vi "Read Params from INI Section.vi"(8 "error in (no error)":errorcluster, 9 "Parameters In":variant, 10 "Refnum in":T1, 11 "Analyze Fluence in":refnum<class "Analyze Fluence.lvclass">) -> (0 "error out":errorcluster, 1 "Parameters Out":variant, 2 "Refnum out":T1, 3 "Analyze Fluence out":refnum<class "Analyze Fluence.lvclass">)   [LabVIEW 2020, in "Analyze.lvlib" / "Analyze Fluence.lvclass"]
uses:
  Analyze Fluence.lvclass
  <vilib>/Utility/config.llb/Config Data RefNum.ctl
  <vilib>/Utility/config.llb/Read Key (Double).vi
  <vilib>/Utility/config.llb/Read Key (I32).vi
  <vilib>/Utility/config.llb/NI_LVConfig.lvlib
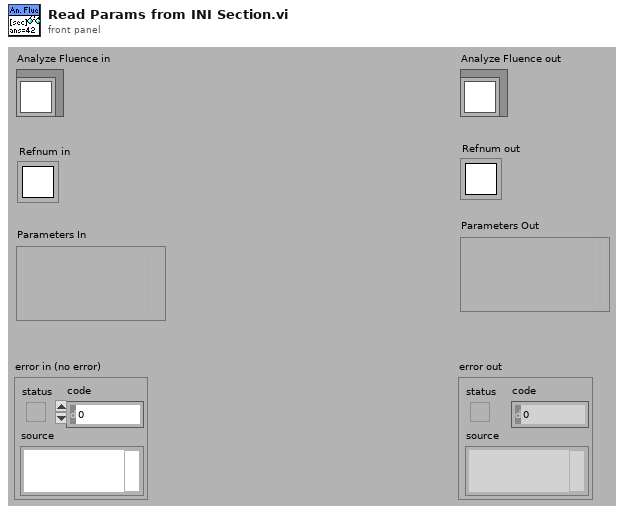
[diagram p1: front panel]
types:
  T1 = typedef "NI_LVConfig.lvlib/Config Data RefNum.ctl" = refnum<k1>
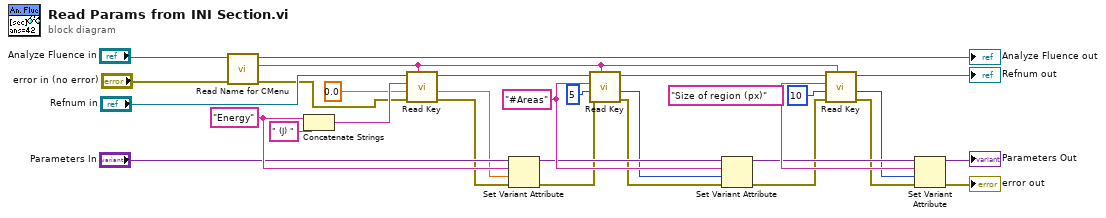
[diagram p0: block diagram]
diagram:
  w30 = "Size of region (px)" ("name")
  w27 = "#Areas" ("name")
  w23 = "Energy" ("name")
  n1 = call-dynamic "Read Name for CMenu.vi"("error in (no error)"="error in (no error)", "Analyze BaseClass in"="Analyze Fluence in") -> ("error out"=w18:errorcluster, "Name for Context menu"=w1:string, "Analyze BaseClass out"=→"Analyze Fluence out":refnum<class "Analyze Fluence.lvclass">)  [unwired: 7 in]
  n2 = Concatenate Strings(w23, " (J) " ("string")) -> (w24:string)
  n3 = call-poly <vilib>:"Read Key.vi"("section"=w1, "error in (no error)"=w18, "default value"=0.0, "key"=w24, "refnum"="Refnum in") -> ("error out"=w6:errorcluster, "value"=w13:dbl, "refnum out"=w26:T1)  [unwired: 3 in, 1 out]
  n4 = Set Variant Attribute(Variant="Parameters In", name=w23, value=w13, error in=w6) -> (Variant out=w22:variant, error out=w5:errorcluster)  [unwired: 1 out]
  n5 = call-poly <vilib>:"Read Key.vi"("section"=w1, "error in (no error)"=w5, "default value"=5, "key"=w27, "refnum"=w26) -> ("error out"=w4:errorcluster, "value"=w14:i32, "refnum out"=w28:T1)  [unwired: 3 in, 1 out]
  n6 = Set Variant Attribute(Variant=w22, name=w27, value=w14, error in=w4) -> (Variant out=w29:variant, error out=w3:errorcluster)  [unwired: 1 out]
  n7 = call-poly <vilib>:"Read Key.vi"("section"=w1, "error in (no error)"=w3, "default value"=10 ("Size of region (px)"), "key"=w30, "refnum"=w28) -> ("error out"=w2:errorcluster, "value"=w10:i32, "refnum out"=→"Refnum out":T1)  [unwired: 3 in, 1 out]
  n8 = Set Variant Attribute(Variant=w29, name=w30, value=w10, error in=w2) -> (Variant out=→"Parameters Out":variant, error out=→"error out":errorcluster)  [unwired: 1 out]
